vi "SDCP SMF Receiver and Transmitter - Rx Table Formatter.vi"(3 "error in (no error)":errorcluster, 4 "Elements of table":T1[](array[typedef]), 5 "Table reference":refnum<vi>) -> (0 "error out":errorcluster)   [LabVIEW 2020]
uses:
  Typedefs/SDCP - Log Table - Element.ctl
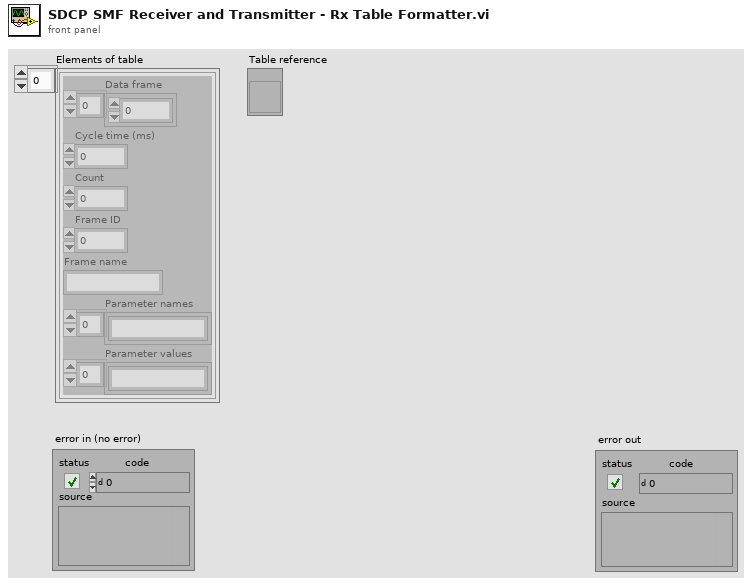
[diagram p1: front panel]
types:
  T1 = typedef "SDCP - Log Table - Element.ctl" = cluster{"Data frame":u8[], "Cycle time (ms)":i32, "Count":i32, "Frame ID":i32, "Frame name":string, "Parameter names":string[], "Parameter values":string[]}
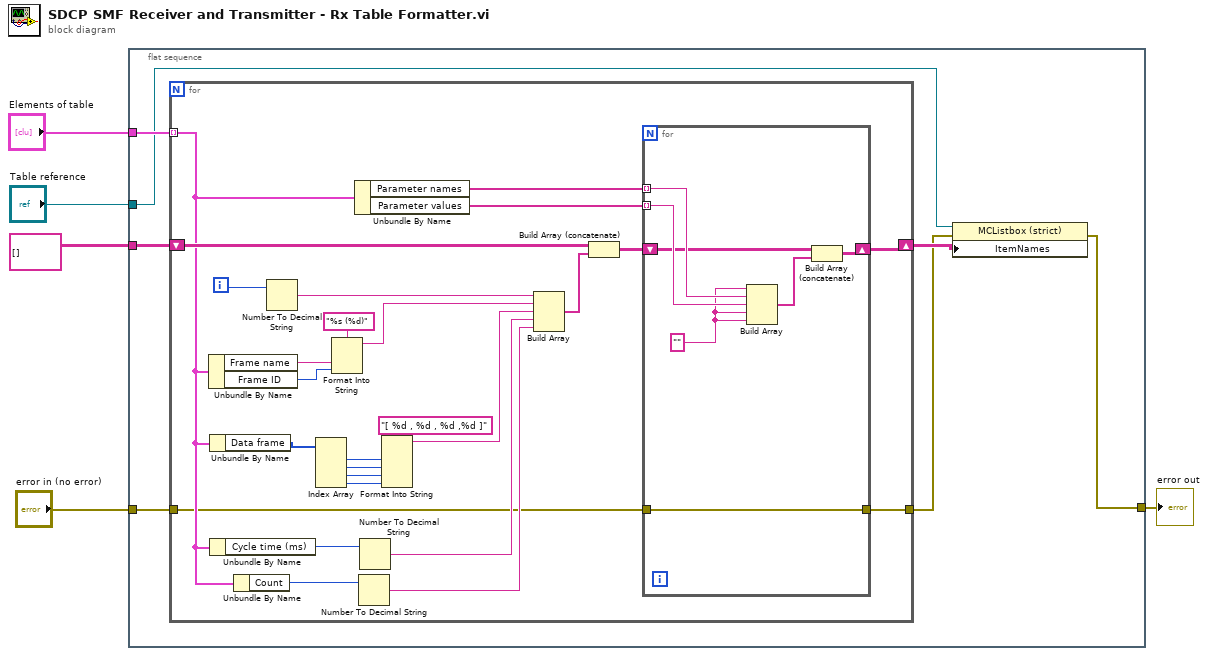
[diagram p0: block diagram]
diagram:
  n1 = flat-sequence {
    tunnel: "error in (no error)" -> [w11]
    tunnel: "Table reference" -> [w9]
    tunnel: "Elements of table" -> [w12]
    tunnel: string[][] [] -> [w10]
    tunnel: [w6] -> w1
    frame #0 {
      n2 = for {
        tunnel: w12 -> [w17] mode=indexing
        tunnel: w11 -> [w14]
        shift-right: [w18] -> w8
        shift-left: w10 -> [w32]
        tunnel: [w13] -> w7
        i -> [w35]
        n3 = Unbundle By Name(w17) -> ("Frame name"=w37:string, "Frame ID"=w36:i32)
        n4 = Unbundle By Name(w17) -> ("Data frame"=w30:u8[])
        n5 = Unbundle By Name(w17) -> ("Cycle time (ms)"=w23:i32)
        n6 = Unbundle By Name(w17) -> ("Count"=w21:i32)
        n7 = Number To Decimal String(number=w35) -> (decimal integer string=w34:string)  [unwired: 1 in]
        n8 = Index Array(array=w30) -> (element #1=w28:u8, element #2=w27:u8, element #3=w26:u8, element #4=w25:u8)  [unwired: 4 in]
        n9 = Format Into String(format string="%s (%d)", w37, w36) -> (resulting string=w33:string)  [unwired: 2 in, 1 out]
        n10 = Unbundle By Name(w17) -> ("Parameter names"=w16:string[], "Parameter values"=w15:string[])
        n11 = Number To Decimal String(number=w21) -> (decimal integer string=w20:string)  [unwired: 1 in]
        n12 = Number To Decimal String(number=w23) -> (decimal integer string=w22:string)  [unwired: 1 in]
        n13 = Format Into String(format string="[ %d , %d , %d ,%d ]", w28, w27, w26, w25) -> (resulting string=w24:string)  [unwired: 2 in, 1 out]
        n14 = Build Array(w34, w33, w24, w22, w20) -> (w31:string[])
        n15 = Build Array (concatenate)(w32, w31) -> (w19:string[][])
        n16 = for {
          shift-right: [w40] -> w18
          shift-left: w19 -> [w42]
          tunnel: w16 -> [w45] mode=indexing
          tunnel: w15 -> [w44] mode=indexing
          tunnel: w14 -> [w39]
          tunnel: [w39] -> w13
          w43 = "" ("element")
          n17 = Build Array(w43, w45, w44, w43, w43) -> (w41:string[])
          n18 = Build Array (concatenate)(w42, w41) -> (w40:string[][])
        }
      }
      n19 = property class="MCListbox (strict)"(reference=w9, error in=w7, "ItemNames"=w8) -> (error out=w6:errorcluster)  [unwired: 1 out]
    }
  }
  "error out" <- w1
